vi "校验码计算.vi"(3 "变量数据":string, 4 "变量地址":string, 5 "读取为0写入为1":string="1") -> (1 "校验码2":string, 2 "校验码1":string)   [LabVIEW 2015, in "PLC.lvlib"]
uses:
  PLC.lvlib
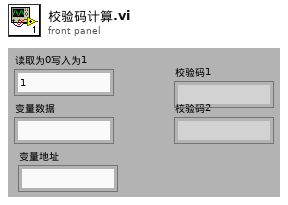
[diagram p1: front panel]
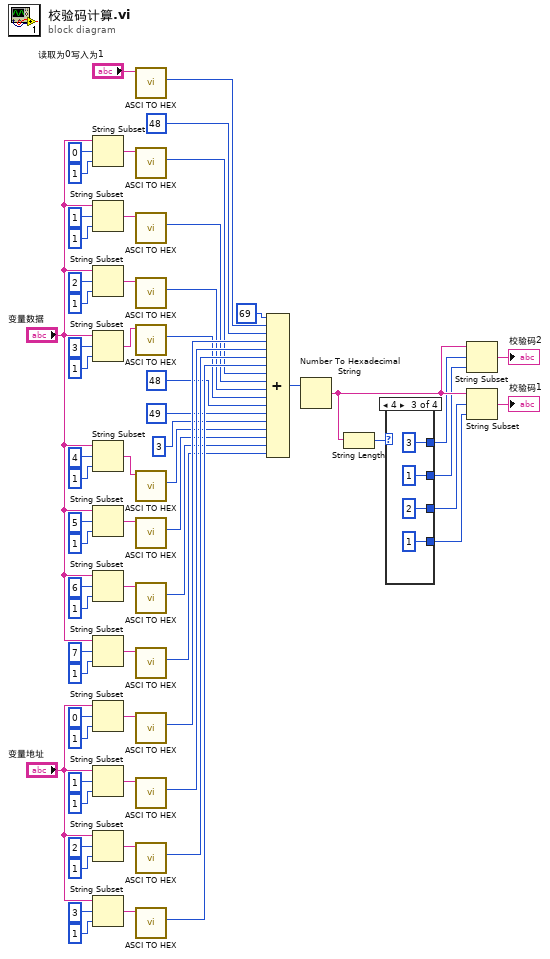
[diagram p0: block diagram]
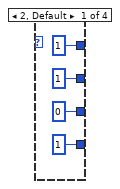
[diagram p2: hidden frame]
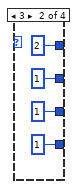
[diagram p3: hidden frame]
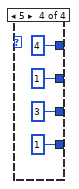
[diagram p4: hidden frame]
diagram:
  n1 = String Subset(string="变量数据", offset (0)=0 ("偏移量(0)"), length (rest)=1 ("长度（剩余）")) -> (substring=w27:string)
  n2 = String Subset(string="变量数据", offset (0)=1 ("偏移量(0)"), length (rest)=1 ("长度（剩余）")) -> (substring=w28:string)
  n3 = String Subset(string="变量数据", offset (0)=2 ("偏移量(0)"), length (rest)=1 ("长度（剩余）")) -> (substring=w29:string)
  n4 = String Subset(string="变量数据", offset (0)=3 ("偏移量(0)"), length (rest)=1 ("长度（剩余）")) -> (substring=w30:string)
  n5 = String Subset(string="变量数据", offset (0)=4 ("偏移量(0)"), length (rest)=1 ("长度（剩余）")) -> (substring=w7:string)
  n6 = String Subset(string="变量数据", offset (0)=5 ("偏移量(0)"), length (rest)=1 ("长度（剩余）")) -> (substring=w8:string)
  n7 = String Subset(string="变量数据", offset (0)=6 ("偏移量(0)"), length (rest)=1 ("长度（剩余）")) -> (substring=w9:string)
  n8 = String Subset(string="变量数据", offset (0)=7 ("偏移量(0)"), length (rest)=1 ("长度（剩余）")) -> (substring=w10:string)
  n9 = String Subset(string="变量地址", offset (0)=0 ("偏移量(0)"), length (rest)=1 ("长度（剩余）")) -> (substring=w59:string)
  n10 = String Subset(string="变量地址", offset (0)=1 ("偏移量(0)"), length (rest)=1 ("长度（剩余）")) -> (substring=w58:string)
  n11 = String Subset(string="变量地址", offset (0)=2 ("偏移量(0)"), length (rest)=1 ("长度（剩余）")) -> (substring=w57:string)
  n12 = String Subset(string="变量地址", offset (0)=3 ("偏移量(0)"), length (rest)=1 ("长度（剩余）")) -> (substring=w56:string)
  n13 = call "ASCI TO HEX.vi"("ASCII"="读取为0写入为1") -> ("数字"=w64:u32)  [unwired: 10 out]
  n14 = call "ASCI TO HEX.vi"("ASCII"=w27) -> ("数字"=w26:u32)  [unwired: 10 out]
  n15 = call "ASCI TO HEX.vi"("ASCII"=w28) -> ("数字"=w25:u32)  [unwired: 10 out]
  n16 = call "ASCI TO HEX.vi"("ASCII"=w29) -> ("数字"=w24:u32)  [unwired: 10 out]
  n17 = call "ASCI TO HEX.vi"("ASCII"=w30) -> ("数字"=w23:u32)  [unwired: 10 out]
  n18 = call "ASCI TO HEX.vi"("ASCII"=w7) -> ("数字"=w5:u32)  [unwired: 10 out]
  n19 = call "ASCI TO HEX.vi"("ASCII"=w8) -> ("数字"=w4:u32)  [unwired: 10 out]
  n20 = call "ASCI TO HEX.vi"("ASCII"=w9) -> ("数字"=w3:u32)  [unwired: 10 out]
  n21 = call "ASCI TO HEX.vi"("ASCII"=w10) -> ("数字"=w2:u32)  [unwired: 10 out]
  n22 = call "ASCI TO HEX.vi"("ASCII"=w59) -> ("数字"=w63:u32)  [unwired: 10 out]
  n23 = call "ASCI TO HEX.vi"("ASCII"=w58) -> ("数字"=w62:u32)  [unwired: 10 out]
  n24 = call "ASCI TO HEX.vi"("ASCII"=w57) -> ("数字"=w61:u32)  [unwired: 10 out]
  n25 = call "ASCI TO HEX.vi"("ASCII"=w56) -> ("数字"=w60:u32)  [unwired: 10 out]
  n26 = Compound Arithmetic op=ADD(u32 69 ("值"), w64, 48 ("长度（剩余）"), w63, w62, w61, w60, w26, w25, w24, w23, 48 ("长度（剩余）"), 49 ("长度（剩余）"), 3 ("值"), w5, w4, w3, w2) -> (w65:u32)
  n27 = Number To Hexadecimal String(2:w65) -> (0:w44:string)  [unwired: 1 out]
  n28 = String Length(string=w44) -> (length=w43:i32)
  n29 = case shown="4" w43 {
    tunnel: [0 ("长度（剩余）") 1 ("偏移量(0)") 2 ("偏移量(0)") 3 ("偏移量(0)")] -> w42
    tunnel: [1 ("长度（剩余）") 1 ("长度（剩余）") 1 ("长度（剩余）") 1 ("长度（剩余）")] -> w41
    tunnel: [1 ("偏移量(0)") 2 ("偏移量(0)") 3 ("偏移量(0)") 4 ("偏移量(0)")] -> w40
    tunnel: [1 ("长度（剩余）") 1 ("长度（剩余）") 1 ("长度（剩余）") 1 ("长度（剩余）")] -> w39
    frame 2, Default {
    }
    frame 3 {
    }
    frame 4 {
    }
    frame 5 {
    }
  }
  n30 = String Subset(string=w44, offset (0)=w40, length (rest)=w39) -> (substring=→"校验码2":string)
  n31 = String Subset(string=w44, offset (0)=w42, length (rest)=w41) -> (substring=→"校验码1":string)
